vi "Append  Monitored Measuremenst to Fit Result.vi"(5 "Channels":string[](array[string]), 6 "Peaks absolute time":dbl[](array[numeric]) format="%#_13g", 7 "Data in":dbl[][](array[numeric]), 8 "Error In":errorcluster, 9 "t group name in":string="t", 10 "mnt group name in":string="mnt", 11 "file path":path=path "C:/Data/test.tdms") -> (0 "Error Out":errorcluster, 2 "Channels out":string[](array[string]), 3 "Data out":dbl[][](array[numeric]))   [LabVIEW 2016]
panel:
  out "Indexes":dbl[][](array[numeric])
  out "mnt time":dbl[](array[numeric]) format="%#_13g"
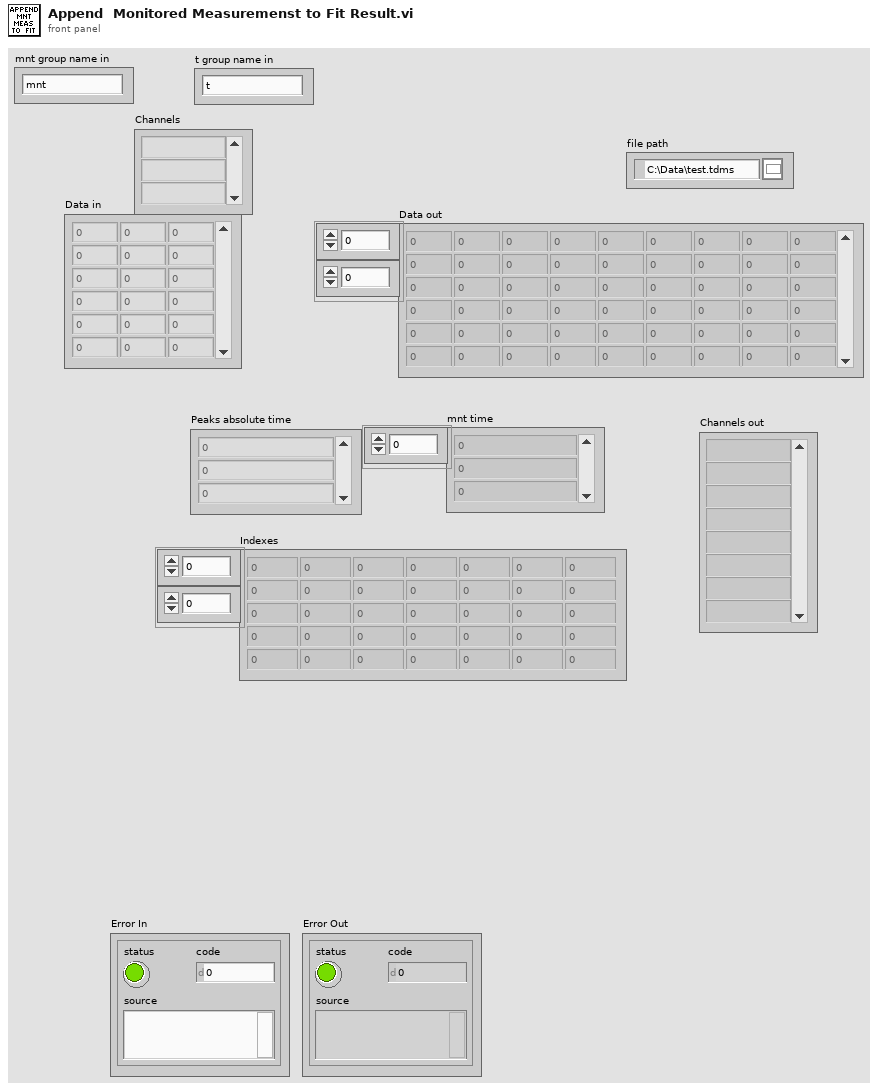
[diagram p1: front panel]
types:
  T1 = enum16{"open", "open or create", "create or replace", "create", "open (read-only)"}
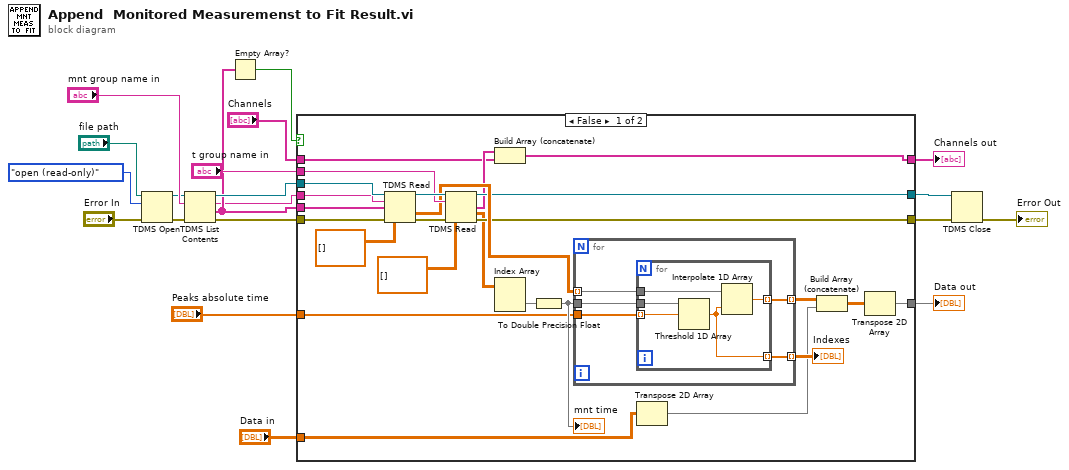
[diagram p0: block diagram]
diagram:
  n1 = TDMS Open(8:"Error In", 10:T1."open (read-only)" ("operation (0:open)"), 11:"file path") -> (0:w15:errorcluster, 3:w14:refnum<k34>)  [unwired: 4 in]
  n2 = TDMS List Contents(4:w15, 6:"mnt group name in", 7:w14) -> (0:w11:errorcluster, 1:w17:string[], 2:w3:string, 3:w18:refnum<k34>)
  n3 = Empty Array?(array=w17) -> (empty?=w8:bool)
  n4 = case shown="False" w8 {
    tunnel: "t group name in" -> [w44 _]
    tunnel: w18 -> [w42 w58]
    tunnel: w17 -> [w41 _]
    tunnel: "Peaks absolute time" -> [w37 _]
    tunnel: w11 -> [w35 w59]
    tunnel: [w34 w59] -> w10
    tunnel: [w33 w58] -> w9
    tunnel: [w26 w57] -> w7
    tunnel: [w25 w56] -> w6
    tunnel: w3 -> [w30 _]
    tunnel: "Data in" -> [w22 w57]
    tunnel: "Channels" -> [w24 w56]
    frame False {
      n5 = TDMS Read(0:w42, 5:w30, 7:w41, 11:w35, 12:dbl[][] []) -> (4:w45:refnum<k34>, 10:w39:dbl[][], 15:w43:errorcluster)  [unwired: 3 in, 3 out]
      n6 = TDMS Read(0:w45, 5:w44, 11:w43, 12:dbl[][] []) -> (4:w33:refnum<k34>, 8:w31:string[], 10:w28:dbl[][], 15:w34:errorcluster)  [unwired: 4 in, 2 out]
      n7 = Build Array (concatenate)(w31, w24) -> (w25:string[])
      n8 = Index Array(array=w28) -> (element=w29:dbl[])  [unwired: 2 in]
      n9 = To Double Precision Float(number=w29) -> (double precision float=w38:dbl[])
      "mnt time" <- w38
      n10 = for {
        tunnel: w39 -> [w48] mode=indexing
        tunnel: w38 -> [w50]
        tunnel: w37 -> [w49]
        tunnel: [w47] -> w32 mode=indexing
        tunnel: [w46] -> w27 mode=indexing
        n11 = for {
          tunnel: w50 -> [w55]
          tunnel: w49 -> [w54] mode=indexing
          tunnel: w48 -> [w53]
          tunnel: [w52] -> w47 mode=indexing
          tunnel: [w51] -> w46 mode=indexing
          n12 = Threshold 1D Array(2:w54, 3:w55) -> (0:w51:dbl)  [unwired: 1 in]
          n13 = Interpolate 1D Array(1:w51, 2:w53) -> (0:w52:dbl)
        }
      }
      "Indexes" <- w27
      n14 = Transpose 2D Array(2D array=w22) -> (transposed array=w21:dbl[][])
      n15 = Build Array (concatenate)(w32, w21) -> (w23:dbl[][])
      n16 = Transpose 2D Array(2D array=w23) -> (transposed array=w26:dbl[][])
    }
    frame True {
    }
  }
  "Channels out" <- w6
  "Data out" <- w7
  n17 = TDMS Close(8:w10, 11:w9) -> (0:→"Error Out":errorcluster)  [unwired: 1 out]
